vi "GenerateCode.vi"(1 "Terms":T1[](array[typedef]), 3 "Diagram":refnum<vi>, 5 "XRef":refnum<vi>, 6 "State In":T4) -> (0 "Generated Code?":bool, 2 "State Out":T4, 4 "Reply":string[](array[string]))   [LabVIEW 2012, in "Array Size and Index.xnode"]
uses:
  Array Size and Index.xnode
  State.ctl
  <vilib>/XNodeSupport/XNodeTermIDPair.ctl
  <vilib>/XNodeSupport/XNodeTermRef.ctl
  <vilib>/XNodeSupport/XNodeString.ctl
  <userlib>/_LAVAcr/Scripting Tools/XNode Support/Find term type by ID_Terminal.vi
  <userlib>/_LAVAcr/Scripting Tools/XNode Support/XNode Support.lvlib
  <userlib>/_LAVAcr/Scripting Tools/Scripting Tools.lvlib
  <vilib>/XNodeSupport/NI_XNodeSupport.lvlib
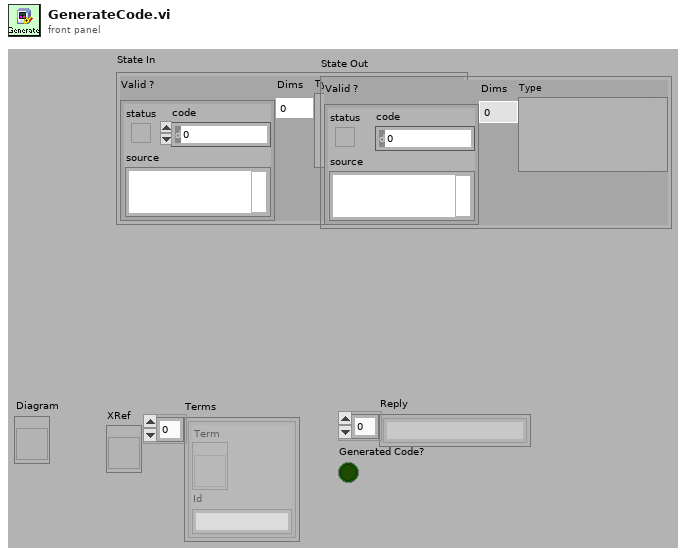
[diagram p1: front panel]
types:
  T1 = typedef "NI_XNodeSupport.lvlib/XNodeTermIDPair.ctl" = cluster{"Term":T2, "Id":T3}
  T2 = typedef "NI_XNodeSupport.lvlib/XNodeTermRef.ctl" = refnum<vi>
  T3 = typedef "NI_XNodeSupport.lvlib/XNodeString.ctl" = string
  T4 = typedef "Array Size and Index.xnode/State.ctl" = cluster{"Valid ?":errorcluster, "Dims":i32, "Type":variant}
  T5 = typedef "NI_XNodeSupport.lvlib/XNodeTermIDPairs.ctl" = T1[]
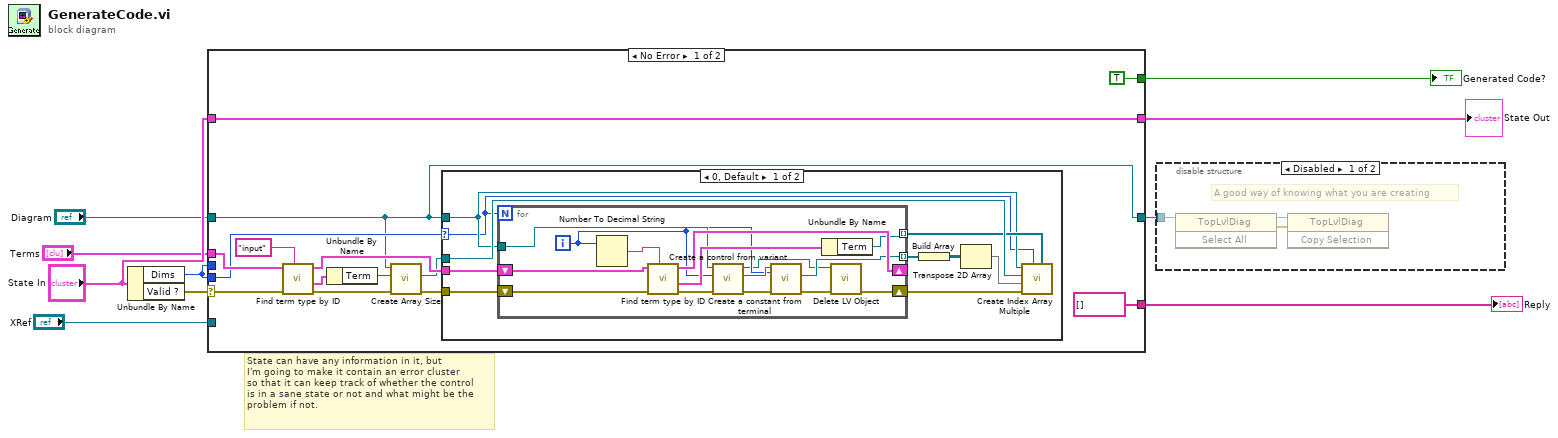
[diagram p0: block diagram]
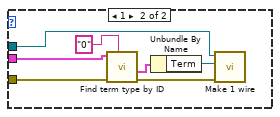
[diagram p2: hidden frame]
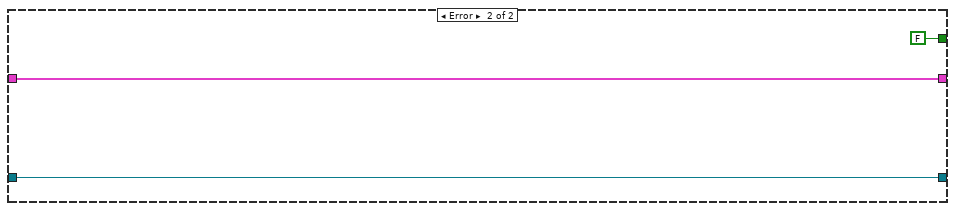
[diagram p3: hidden frame]
diagram:
  # "State can have any information in it, but\nI'm going to make it contain an error cluster\nso that it can keep track of whether the control\nis in a sane state or not and what might be the\nproblem if not."
  n1 = Unbundle By Name("State In") -> ("Dims"=w1:i32, "Valid ?"=w10:errorcluster)
  n2 = case shown="No Error" w10 {
    selector: w10 -> [w16 _]
    tunnel: "State In" -> [w22 w59]
    tunnel: "Diagram" -> [w11 w57]
    tunnel: "Terms" -> [w20 _]
    tunnel: "XRef" -> [_ _]
    tunnel: [w11 w57] -> w3
    tunnel: [string[] [] ("Reply") _] -> w6
    tunnel: [TRUE FALSE] -> w5
    tunnel: [w22 w59] -> w4
    tunnel: w1 -> [_ _]
    tunnel: w1 -> [w15 _]
    frame No Error {
      n3 = call-poly <userlib>:"Find term type by ID.vi"("Search ID"="input", "error in (no error)"=w16, "Term Types"=w20) -> ("error out"=w17:errorcluster, "Terminal"=w19:T1, "Other Term Types"=w13:T5)  [unwired: 6 out]
      n4 = Unbundle By Name(w19) -> ("Term"=w18:T2)
      n5 = call <userlib>:"Create Array Size.vi"("error in (no error)"=w17, "Source"=w18, "Diagram In"=w11) -> ("error out"=w14:errorcluster, "Output Terminal"=w12:refnum<vi>)  [unwired: 2 in, 5 out]
      n6 = case shown="0, Default" w15 {
        selector: w15 -> [w26 _]
        tunnel: w14 -> [w30 w55]
        tunnel: w13 -> [w33 w54]
        tunnel: w12 -> [w34 w50]
        tunnel: w11 -> [w31 _]
        frame 0, Default {
          n7 = for {
            N: w26 -> [_]
            shift-right: [w48] -> _
            shift-left: w33 -> [w49]
            tunnel: [w45] -> w32 mode=indexing
            tunnel: w31 -> [w44]
            shift-right: [w37] -> w27
            shift-left: w30 -> [w42]
            tunnel: [w38] -> w29 mode=indexing
            i -> [w39]
            n8 = Number To Decimal String(number=w39) -> (decimal integer string=w47:string)  [unwired: 1 out]
            n9 = call-poly <userlib>:"Find term type by ID.vi"("Search ID"=w47, "error in (no error)"=w42, "Term Types"=w49) -> ("error out"=w43:errorcluster, "Terminal"=w46:T1, "Other Term Types"=w48:T5)  [unwired: 6 out]
            n10 = call <userlib>:"Create a control from variant.vi"("error in (no error)"=w43, "Constant Data"=w39, "Diagram"=w44) -> ("error out"=w41:errorcluster, "Terminal"=w40:refnum<vi>, "Control Reference"=w35:refnum<vi>)  [unwired: 4 in, 2 out]
            n11 = call <userlib>:"Create a constant from terminal.vi"("error in (no error)"=w41, "Value"=w39, "Constant from this terminal"=w40) -> ("error out"=w36:errorcluster, "Terminal"=w38:refnum<vi>)  [unwired: 1 in, 6 out]
            n12 = Unbundle By Name(w46) -> ("Term"=w45:T2)
            n13 = call <userlib>:"Delete LV Object.vi"("error out 2"=w36, "reference"=w35) -> ("error out"=w37:errorcluster)  [unwired: 8 out]
          }
          n14 = Build Array(w29) -> (w28:refnum<vi>[][])
          n15 = Transpose 2D Array(2D array=w28) -> (transposed array=w25:refnum<vi>[][])
          n16 = call <userlib>:"Create Index Array Multiple.vi"("Sink"=w32, "Index Count"=w26, "error in (no error)"=w27, "Index"=w25, "Array"=w34, "Diagram In"=w31) -> ()  [unwired: 1 in, 5 out]
        }
        frame 1 {
          n17 = call-poly <userlib>:"Find term type by ID.vi"("Search ID"="0", "error in (no error)"=w55, "Term Types"=w54) -> ("error out"=w56:errorcluster, "Terminal"=w52:T1)  [unwired: 7 out]
          n18 = Unbundle By Name(w52) -> ("Term"=w51:T2)
          n19 = call <userlib>:"Make 1 wire.vi"("error in"=w56, "Wire Terminal 2"=w51, "Wire Terminal 1"=w50) -> ()  [unwired: 9 out]
        }
      }
    }
    frame Error {
    }
  }
  "State Out" <- w4
  "Reply" <- w6
  "Generated Code?" <- w5
  n20 = disable-structure shown="Disabled" {
    disable-tunnel: w3 -> [w60 _]
    frame Disabled {
      # "A good way of knowing what you are creating"
      n21 = invoke class="TopLvlDiag" method="Select All"(reference=w60) -> (reference out=w62:refnum<vi>, error out=w61:errorcluster)  [unwired: 2 in, 1 out]
      n22 = invoke class="TopLvlDiag" method="Copy Selection"(reference=w62, error in=w61) -> ()  [unwired: 1 in, 3 out]
    }
    frame Enabled {
    }
  }
